vi "Gyro PID Fwd Color Assisted.vi"(6 "Target angle":sgl, 7 "Threshold to Color":i32=1200, 8 "Threshold to slow":i32=1000, 9 "Min. speed":i32=40, 10 "Max. speed":i32=80, 11 "EV3 in":T1) -> (3 "EV3 out":T1)   [LabVIEW 2016]
uses:
  <vilib>/NXT/Subs/LVHSConnector.ctl
  <vilib>/NXT/LegoClasses/BrickReference/BrickReference.lvclass
  <vilib>/NXT/Block Support/NXT_OutputPort.ctl
  <vilib>/NXT/Block Support/NXT_InputPort.ctl
  <vilib>/NXT/NXTIO Xnodes/NXTIONodeSubVIs/LEGOResetMotors.vi
  <vilib>/NXT/Dual Mode Library/Motors/Rotation.vi
  <vilib>/NXT/Dual Mode Library/Sensors/EV3_Color_Reflect.vi
  <vilib>/NXT/NXTIO Xnodes/NXTIONodeSubVIs/NXTMotorSteeringOn.vi
  <vilib>/NXT/NXTIO Xnodes/NXTIONodeSubVIs/NXTStopMotors.vi
  <vilib>/NXT/Dual Mode Library/Waits/Wait_Num.vi
  <vilib>/NXT/NXTIO Xnodes/NXTIOXNode/NXTIO.xnode
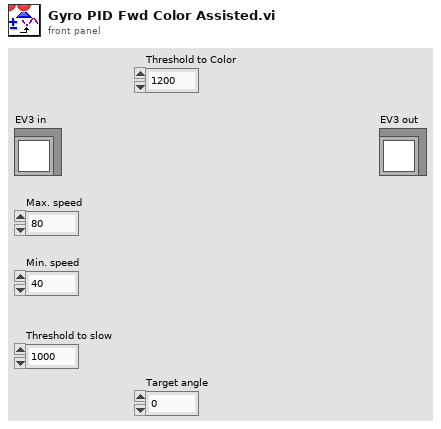
[diagram p1: front panel]
types:
  T1 = typedef "LVHSConnector.ctl" = refnum<class "BrickReference.lvclass">
  T2 = typedef "NXT_OutputPort.ctl" = u8
  T3 = typedef "NXT_InputPort.ctl" = u32
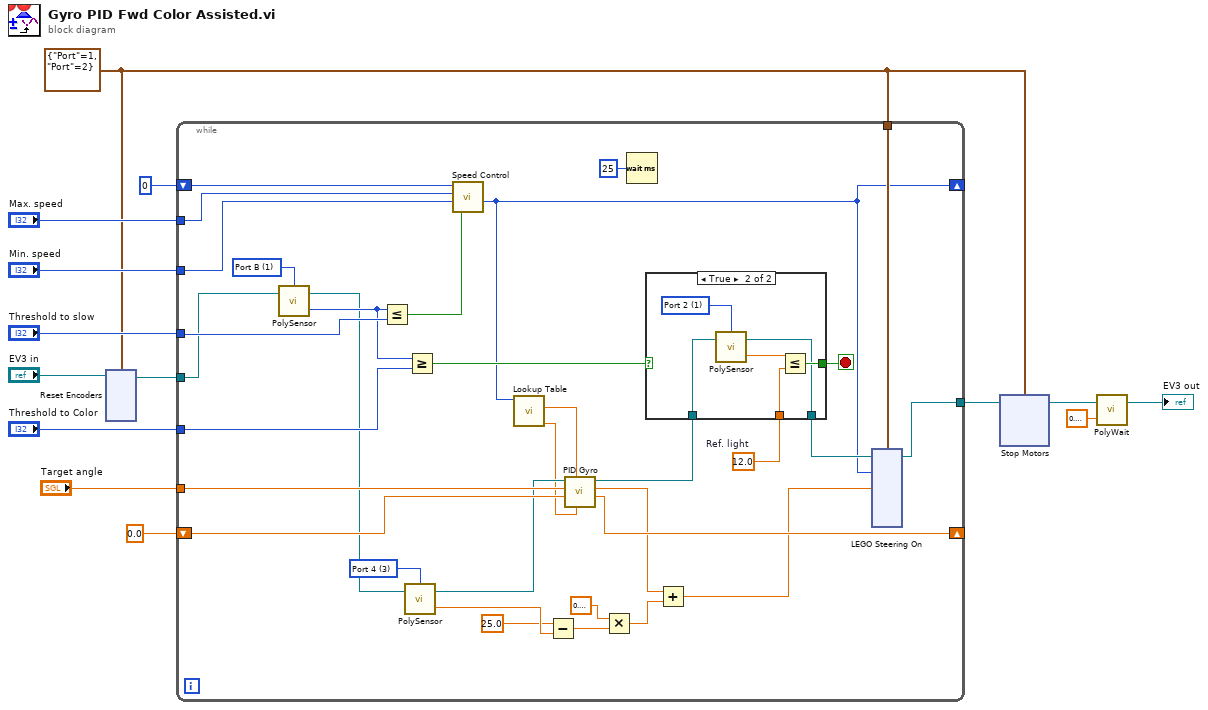
[diagram p0: block diagram]
diagram:
  w4 = cluster{"Port":T2, "Port":T2} {"Port"=1, "Port"=2} ("Motor")
  n1 = xnode "Reset Encoders"("Motors"=w4, "NXT/EV3"="EV3 in") -> ("NXT/EV3"=w10:T1)
  n2 = while {
    tunnel: w10 -> [w37]
    shift-right: [w47] -> _
    shift-left: sgl 0.0 -> [w34]
    tunnel: "Target angle" -> [w46]
    tunnel: [w43] -> w6
    tunnel: w4 -> [w45]
    shift-right: [w17] -> _
    shift-left: 0 -> [w41]
    tunnel: "Min. speed" -> [w38]
    tunnel: "Max. speed" -> [w40]
    tunnel: "Threshold to slow" -> [w39]
    tunnel: "Threshold to Color" -> [w33]
    stop <- w32 stop-if-true
    w27 = T3 3 items=["Port 1", "Port 2", "Port 3", "Port 4"] ("Port (Port 1)")
    w28 = sgl 12.0  # Ref. light
    w44 = T2 1 items=["Port A", "Port B", "Port C", "Port D"] ("Port (Port A)")
    n3 = call-poly <vilib>:"PolySensor.vi"("NXT/EV3"=w37, "Port (Port A)"=w44) -> ("Angle of Rotation"=w35:i32, "NXT/EV3"=w26:T1)  [unwired: 1 in]
    n4 = Less Or Equal?(x=w35, y=w39) -> (x <= y?=w36:bool)
    n5 = call-poly <vilib>:"PolySensor.vi"("NXT/EV3"=w26, "Port (Port 1)"=w27) -> ("Scaled Value"=w19:sgl, "NXT/EV3"=w25:T1)  [unwired: 1 in]
    n6 = Greater Or Equal?(x=w35, y=w33) -> (x >= y?=w31:bool)
    n7 = call "Speed Control.vi"("Speed Up or Down?"=w36, "Min. speed"=w38, "Max. speed"=w40, "Ini. speed"=w41) -> ("Speed out"=w17:i32)  [unwired: 7 in]
    n8 = call "Lookup Table.vi"("Speed"=w17) -> ("I"=w15:dbl, "P"=w16:dbl)  [unwired: 9 in]
    n9 = Subtract(x=sgl 25.0 ("y"), y=w19) -> (x-y=w24:sgl)
    n10 = call "PID Gyro.vi"("K_i"=w15, "K_p"=w16, "Previous integral"=w34, "Target angle"=w46, "EV3 in"=w25) -> ("New integral"=w47:sgl, "Total error"=w21:sgl, "EV3 out"=w30:T1)  [unwired: 4 in]
    n11 = Multiply(x=sgl 0.3, y=w24) -> (x*y=w22:sgl)
    n12 = Wait (ms)(milliseconds to wait=u32 25) -> ()  [unwired: 1 out]
    n13 = case shown="True" w31 {
      tunnel: [_ w52] -> w32
      tunnel: w30 -> [w48 w51]
      tunnel: [w48 w50] -> w29
      tunnel: w28 -> [_ w49]
      frame False {
      }
      frame True {
        w54 = T3 1 items=["Port 1", "Port 2", "Port 3", "Port 4"] ("Port (Port 1)")
        n14 = call-poly <vilib>:"PolySensor.vi"("NXT/EV3"=w51, "Port (Port 1)"=w54) -> ("Scaled Value"=w53:sgl, "NXT/EV3"=w50:T1)  [unwired: 1 in]
        n15 = Less Or Equal?(x=w53, y=w49) -> (x <= y?=w52:bool)
      }
    }
    n16 = Add(x=w21, y=w22) -> (x+y=w20:sgl)
    n17 = xnode "LEGO Steering On"("Steering 1"=w20, "Power 1"=w17, "Motors"=w45, "NXT/EV3"=w29) -> ("NXT/EV3"=w43:T1)
  }
  n18 = xnode "Stop Motors"("Motors"=w4, "NXT/EV3"=w6) -> ("NXT/EV3"=w5:T1)
  n19 = call-poly <vilib>:"PolyWait.vi"("Time (1 sec)"=sgl 0.2, "NXT/EV3"=w5) -> ("NXT/EV3"=→"EV3 out":T1)  [unwired: 2 in]
